vi "Run Refill.vi"(8 "error in (no error)":errorcluster, 9 "auto_switch_valve":bool=TRUE, 10 "flow_rate_uL_s":dbl=200.0, 11 "PHD Ultra in":refnum<class "PHD Ultra.lvclass">) -> (0 "error out":errorcluster, 3 "PHD Ultra out":refnum<class "PHD Ultra.lvclass">)   [LabVIEW 2018, in "PHD Ultra.lvlib" / "PHD Ultra.lvclass"]
uses:
  PHD Ultra.lvclass
  <userlib>/QmixLib/QmixLib.lvlib
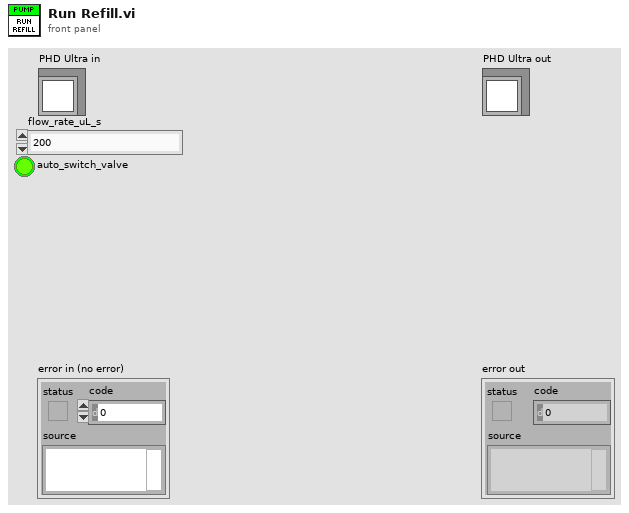
[diagram p1: front panel]
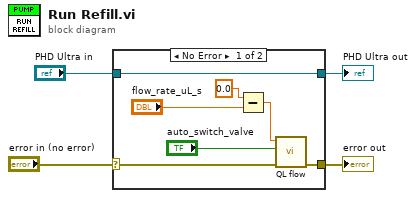
[diagram p0: block diagram]
diagram:
  n1 = case shown="No Error" "error in (no error)" {
    selector: "error in (no error)" -> [w10 w13]
    tunnel: [w9 w13] -> w3
    tunnel: [w11 w12] -> w1
    tunnel: "PHD Ultra in" -> [w11 w12]
    frame No Error {
      n2 = Subtract(x=0.0, y="flow_rate_uL_s") -> (x-y=w7:dbl)
      n3 = call <userlib>:"QL flow.vi"("error in (no error)"=w10, "auto_switch_valve"="auto_switch_valve", "flow_rate_uL_s"=w7) -> ("error out"=w9:errorcluster)  [unwired: 8 in]
    }
    frame Error {
    }
  }
  "error out" <- w3
  "PHD Ultra out" <- w1
